vi "SoftAP Config Test.vi"() -> ()   [LabVIEW 2014, in "ESP8266 WiFi Wrapper.lvlib"]
uses:
  <vilib>/Aledyne-TSXperts/Arduino Compatible Compiler for LabVIEW/addons/ESP8266 WiFi Wrapper/ESP8266 WiFi Wrapper.lvlib
panel:
  in  "DNS address":u8[](array[numeric])=[1, 2, 3, 4]
  in  "IP address":u8[](array[numeric])=[192, 168, 0, 5]
  in  "Gateway address":u8[](array[numeric])=[192, 168, 0, 1]
  in  "Subnet mask":u8[](array[numeric])=[255, 255, 255, 0]
  out "Error Out":errorcluster
  in  "Error In":errorcluster
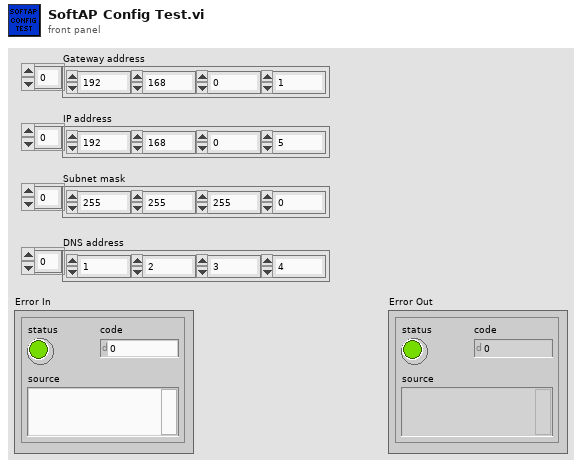
[diagram p1: front panel]
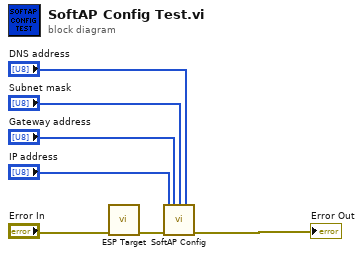
[diagram p0: block diagram]
diagram:
  n1 = call <vilib>:"ESP Target.vi"("Error In"="Error In") -> ("Error Out"=w3:errorcluster)  [unwired: 10 in]
  n2 = call <vilib>:"SoftAP Config.vi"("IP address"="IP address", "Gateway address"="Gateway address", "Subnet mask"="Subnet mask", "DNS address"="DNS address", "Error In"=w3) -> ("Error Out"=→"Error Out":errorcluster)  [unwired: 10 in]
